vi "NIDCPower_channel_ganging - initiate.vi"(8 "error in (no error)":errorcluster, 11 "Ganged Session In":T1) -> (0 "error out":errorcluster, 3 "Ganged Session Out":T1)   [LabVIEW 2024]
uses:
  ctl/NIDCPower_channel_ganging - ctl - ganged session.ctl
  ctl/NIDCPower_channel_ganging - ctl - ganged config.ctl
  ctl/NIDCPower_channel_ganging - ctl - channel mode.ctl
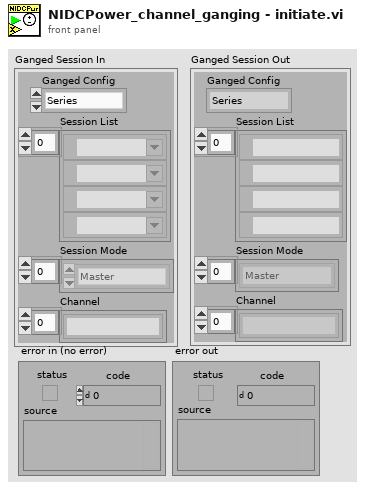
[diagram p1: front panel]
types:
  T1 = typedef "NIDCPower_channel_ganging - ctl - ganged session.ctl" = cluster{"Ganged Config":T2, "Session List":refnum<k15>[], "Session Mode":T3[], "Channel":string[]}
  T2 = typedef "NIDCPower_channel_ganging - ctl - ganged config.ctl" = enum32{"Series", "Parallel", "Manual"}
  T3 = typedef "NIDCPower_channel_ganging - ctl - channel mode.ctl" = enum32{"Master", "Slave", "Slave - Inverted"}
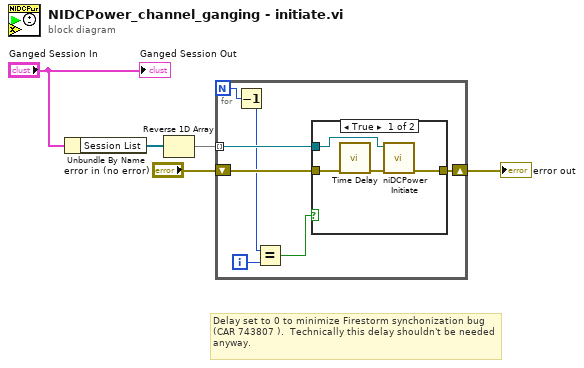
[diagram p0: block diagram]
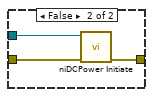
[diagram p2: hidden frame]
diagram:
  # "Delay set to 0 to minimize Firestorm synchonization bug (CAR 743807 ).  Technically this delay shouldn't be needed anyway."
  n1 = Unbundle By Name("Ganged Session In") -> ("Session List"=w1:refnum<k15>[])
  n2 = Reverse 1D Array(array=w1) -> (reversed array=w3:refnum<k15>[])
  n3 = for {
    N -> [w8]
    shift-right: [w10] -> w4
    shift-left: "error in (no error)" -> [w12]
    tunnel: w3 -> [w11] mode=indexing
    i -> [w9]
    n4 = Decrement(x=w8) -> (x-1=w7:i32)
    n5 = Equal?(x=w7, y=w9) -> (x = y?=w6:bool)
    n6 = case shown="True" w6 {
      tunnel: w12 -> [w15 w19]
      tunnel: w11 -> [w13 w18]
      tunnel: [w16 w17] -> w10
      frame True {
        n7 = call "Time Delay"("error in (no error)"=w15) -> ("error out"=w14:errorcluster)  [unwired: 10 in]
        n8 = call <instrlib>:"niDCPower Initiate.vi"("error in (no error)"=w14, "instrument handle"=w13) -> ("error out"=w16:errorcluster)  [unwired: 8 in, 1 out]
      }
      frame False {
        n9 = call <instrlib>:"niDCPower Initiate.vi"("error in (no error)"=w19, "instrument handle"=w18) -> ("error out"=w17:errorcluster)  [unwired: 8 in, 1 out]
      }
    }
  }
  "error out" <- w4
  "Ganged Session Out" <- "Ganged Session In"
